vi "RSZVB Select Admitances.vi"(6 "Out Port (1)":i32=1, 7 "In Port (1)":i32=1, 8 "error in (no error)":errorcluster {"code" format="%.0x"}, 9 "Trace Name (Trc1)":string="Trc1", 10 "Channel (1)":i32=1, 11 "VISA session":refnum<visa-resource-name>) -> (0 "error out":errorcluster {"code" format="%.0x"}, 3 "dup VISA session":refnum<visa-resource-name>)   [LabVIEW 2011]
doc: "This VI select the 2-port (or more ports) converted matched-circuit admittance parameters. The parameters describe the admittances of a 2-port (or more ports) DUT, obtained in forward and reverse transmission and reflection measurements:\n\nY11 is the input admittance of a 2-port DUT that is terminated at its output with the reference impedance Z0 (matched-circuit admittance measured in a forward reflection measurement).\n\nY22 is the output admittance of a 2-port DUT that is terminated at its input with the reference impedance Z0 (matched-circuit admittance measured in a reverse reflection measurement).\n\nY12 and Y21 denote the forward and reverse transfer admittances, respectively.\n\nThe analyzer can also provide matched-circuit admittances for more drive ports or balanced port configurations.\n\nAssigns a measurement parameter to an existing trace or creates a trace and assigns a channel number, a name and a measurement parameter to it. The trace is not displayed.\n\nThe notation for converted admittance parameters and the VIality is analogous to the definition of S-parameters.\n\nRemote-control command(s):\nCALCulate<Ch>:PARameter:SDEFine '<string>', 'Y-S11' | 'Y-S12' | 'Y-S21' | 'Y-S22' | ...\nCALCulate<Ch>:PARameter:MEASure '<string>', 'Y-S11' | 'Y-S12' | 'Y-S21' | 'Y-S22' | ..."
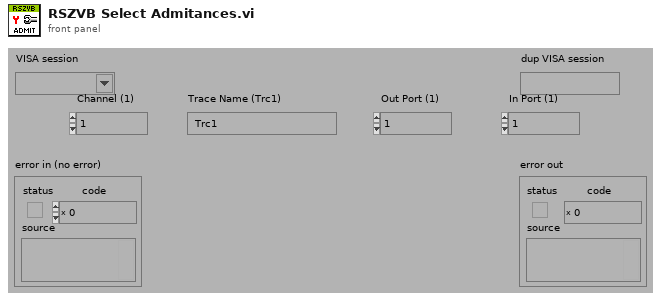
[diagram p1: front panel]
types:
  T1 = cluster{"Error Checking (T: On)":bool, "Installed Options":string[], "Data Valid?":bool, "Ports":i32, "Model":string[], "Option Checking (T: On)":bool}
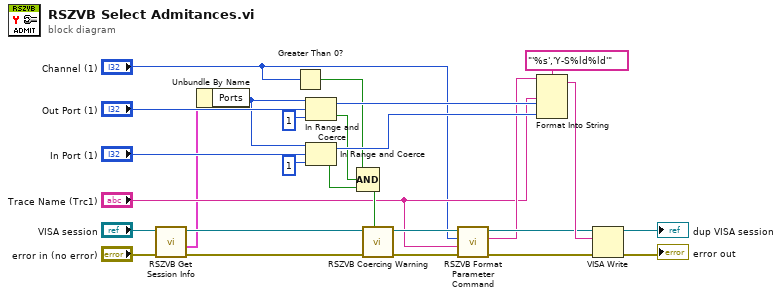
[diagram p0: block diagram]
diagram:
  n1 = call "RSZVB Get Session Info.vi"("error in (no error)"="error in (no error)", "VISA session"="VISA session") -> ("error out"=w4:errorcluster, "Session Info"=w2:T1, "dup VISA session"=w3:refnum<visa-resource-name>)  [unwired: 7 in]
  n2 = Unbundle By Name(w2) -> ("Ports"=w1:i32)
  n3 = Greater Than 0?(x="Channel (1)") -> (x > 0?=w23:bool)
  n4 = In Range and Coerce(upper limit=w1, x="Out Port (1)", lower limit=1) -> (coerced(x)=w24:i32, In Range?=w14:bool)
  n5 = In Range and Coerce(upper limit=w1, x="In Port (1)", lower limit=1) -> (coerced(x)=w26:i32, In Range?=w13:bool)
  n6 = Compound Arithmetic op=AND(w23, w14, w13) -> (w22:bool)
  n7 = call "RSZVB Coercing Warning.vi"("In Range?"=w22, "error in (no error)"=w4, "VISA session"=w3) -> ("error out"=w19:errorcluster, "dup VISA session"=w18:refnum<visa-resource-name>)  [unwired: 7 in]
  n8 = call "RSZVB Format Parameter Command.vi"("error in (no error)"=w19, "Trace Name (Trc1)"="Trace Name (Trc1)", "Channel (1)"="Channel (1)", "VISA session"=w18) -> ("error out"=w20:errorcluster, "Buffer"=w15:string, "dup VISA session"=w17:refnum<visa-resource-name>)  [unwired: 5 in]
  n9 = Format Into String(format string="'%s','Y-S%ld%ld'", initial string=w15, "Trace Name (Trc1)", w24, w26) -> (resulting string=w21:string)  [unwired: 1 in, 1 out]
  n10 = VISA Write(VISA resource name=w17, write buffer=w21, error in (no error)=w20) -> (VISA resource name out=→"dup VISA session":refnum<visa-resource-name>, error out=→"error out":errorcluster)  [unwired: 1 out]
